vi "Main example.vi"() -> ()   [LabVIEW 2020]
uses:
  Control PaP/Support/Move motor.ctl
  Public/Controls/Command to motor.ctl
  Example States.ctl
  Control PaP/Support/Channel configuration--cluster.ctl
  Control PaP/Libraries/NI DAQ/NI DAQ.lvlib
  Control PaP/Libraries/TDS1002 Oscilloscope/TDS1002 Oscilloscope.lvlib
  <resource>/objmgr/daqmx.rc
  Control de MaP.lvlib
panel:
  in  "Motor params":T1={"Tipo"=0, "Dirección"=0, "N°. Pasos"=200, "Frecuencia (Hz)"=255, "Tipo de paso"=1} caption="Parámetros del motor" {"Tipo de paso" items=["Medio paso", "Paso completo"]; "Dirección" items=["Izquierda", "Derecha"]; "Tipo" items=["Unipolar", "Bipolar"]}
  out "Waveform Graph":waveform(dbl)(graph)
  in  "Mover motor":T2
  in  "Driver de motor":refnum<visa-resource-name>
  in  "Osciloscopio":refnum<visa-resource-name>
  in  "DAQ":u16(ring) items=["DAQ_Simulada", "Dev1"]
  in  "stop":bool
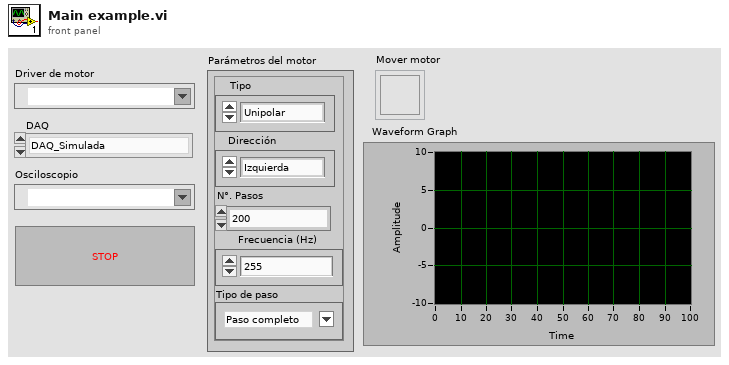
[diagram p1: front panel]
types:
  T1 = typedef "Control de MaP.lvlib/Command to motor.ctl" = cluster{"Tipo":u8, "Dirección":u8, "N°. Pasos":u16, "Frecuencia (Hz)":u8, "Tipo de paso":u8}
  T2 = typedef "Move motor.ctl" = bool
  T3 = cluster{"Driver de motor":refnum<visa-resource-name>, "DAQ ID":i32, "TDS ID":i32}
  T4 = typedef "Example States.ctl" = enum16{"Wait", "Initialize", "Exit"}
  T5 = typedef "TDS1002 Oscilloscope.lvlib/Broadcast Events--cluster.ctl" = cluster{"Module Did Init":refnum<user-event>, "Status Updated":refnum<user-event>, "Error Reported":refnum<user-event>, "Module Did Stop":refnum<user-event>, "Update Module Execution Status":refnum<user-event>, "Helper Loop Status Updated":refnum<user-event>, "Device connected":refnum<user-event>, "Device disconnected":refnum<user-event>, "Data acquired":refnum<user-event>}
  T6 = typedef "NI DAQ.lvlib/Broadcast Events--cluster.ctl" = cluster{"Module Did Init":refnum<user-event>, "Status Updated":refnum<user-event>, "Error Reported":refnum<user-event>, "Module Did Stop":refnum<user-event>, "Update Module Execution Status":refnum<user-event>, "Data acquired":refnum<user-event>}
  T7 = enum16{"All", "DO task", "DI task", "AO task", "AI task"}
  T8 = typedef "TDS1002 Oscilloscope.lvlib/Channel configuration--cluster.ctl" = cluster{"Acquisition Type":i32, "Averaged Waveforms":i32, "Channel":i32, "Probe Attenuation":i32}
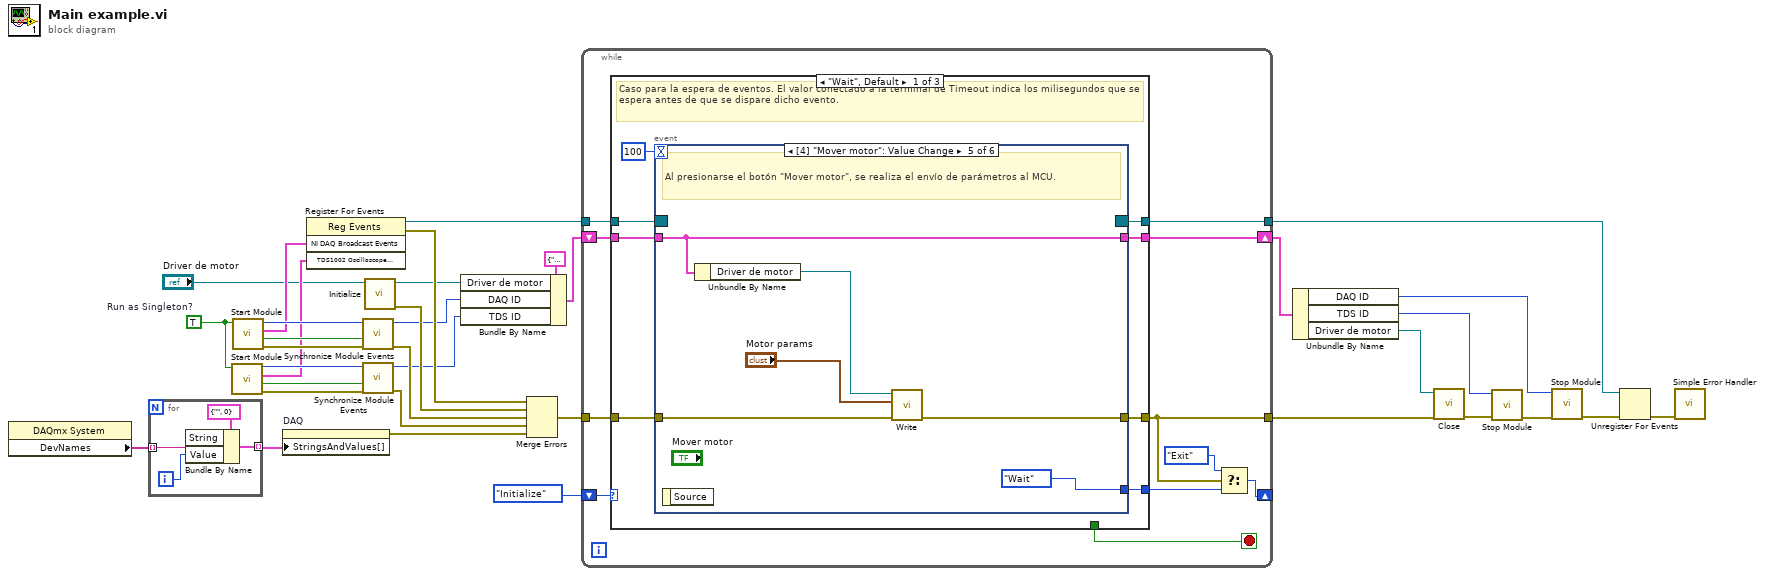
[diagram p0: block diagram]
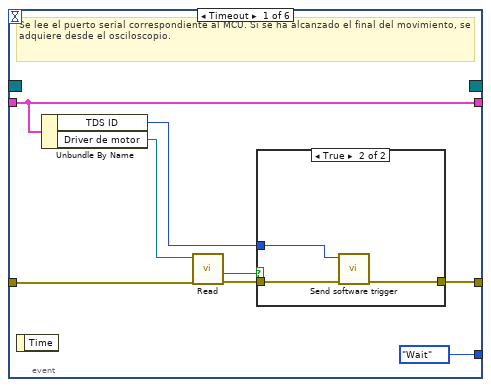
[diagram p2: hidden frame]
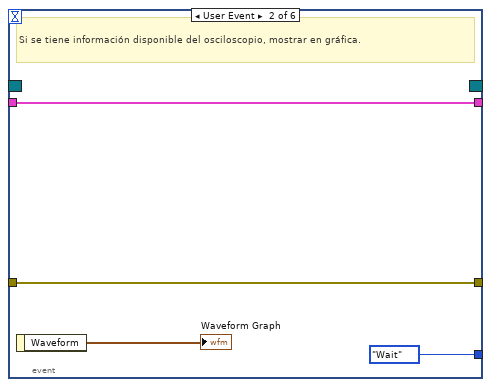
[diagram p4: hidden frame]
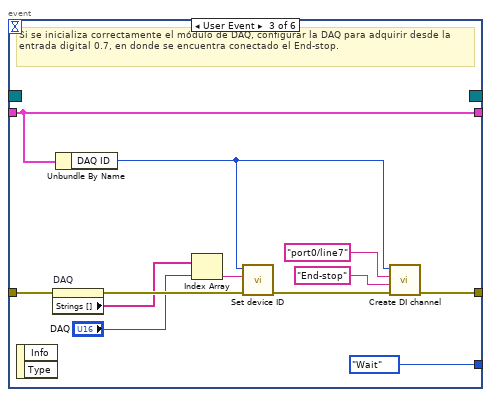
[diagram p5: hidden frame]
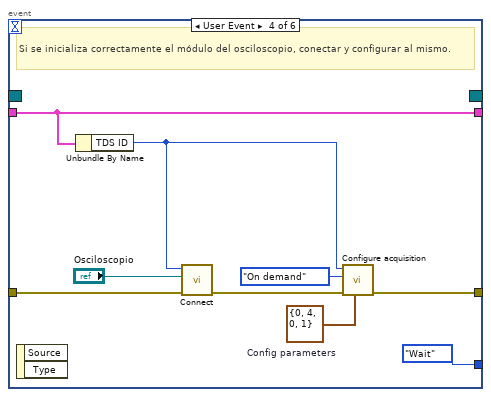
[diagram p6: hidden frame]
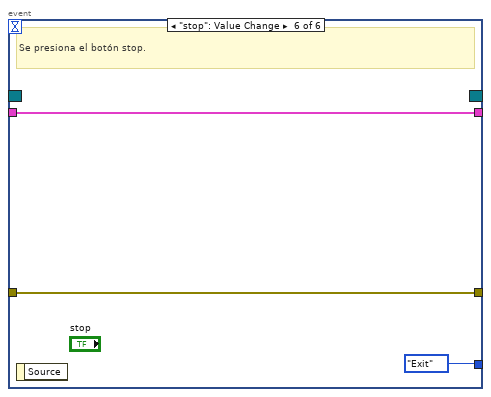
[diagram p7: hidden frame]
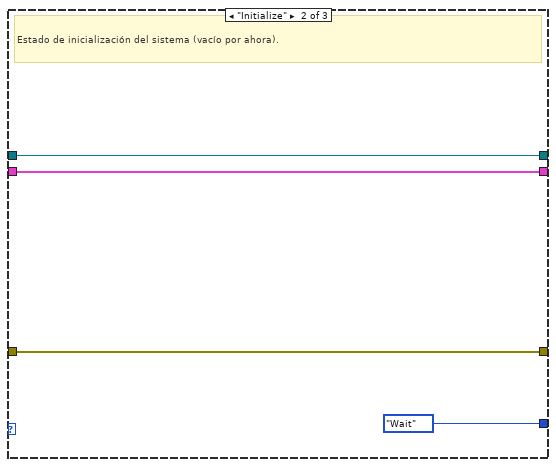
[diagram p8: hidden frame]
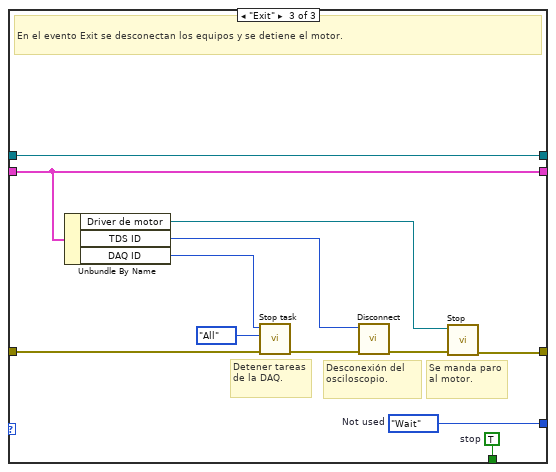
[diagram p9: hidden frame]
diagram:
  w23 = TRUE  # Run as Singleton?
  n1 = property class="DAQmx System"() -> ("DevNames"=w2:tag[])  [unwired: 2 in, 2 out]
  n2 = for {
    tunnel: w2 -> [w38] mode=indexing
    tunnel: [w36] -> w3 mode=indexing
    i -> [w37]
    n3 = Bundle By Name(cluster=cluster{"String":string, "Value":u16} {"String"="", "Value"=0} ("Cluster"), "String"=w38, "Value"=w37) -> (w36:cluster{"String":string, "Value":u16})
  }
  n4 = call "Start Module.vi"("Run as Singleton? (F)"=w23) -> ("error out"=w32:errorcluster, "Wait for Event Sync?"=w30:bool, "TDS1002 Oscilloscope Broadcast Events"=w28:T5, "Module ID"=w31:i32)  [unwired: 7 in]
  n5 = call "Start Module.vi"("Run as Singleton? (F)"=w23) -> ("error out"=w35:errorcluster, "Wait for Event Sync?"=w33:bool, "NI DAQ Broadcast Events"=w29:T6, "Module ID"=w34:i32)  [unwired: 7 in]
  n6 = property on="DAQ" class="Ring (strict)"("StringsAndValues[]"=w3) -> (error out=w1:errorcluster)  [unwired: 2 in, 1 out]
  n7 = register-events(w29, w28) -> (reference out=w20:refnum<event-registration>, error out=w25:errorcluster)  [unwired: 2 in]
  n8 = call "Synchronize Module Events.vi"("error in"=w35, "Wait for Event Sync?"=w33, "Module ID in"=w34) -> ("error out"=w26:errorcluster, "Module ID out"=w12:i32)  [unwired: 7 in]
  n9 = call "Synchronize Module Events.vi"("error in"=w32, "Wait for Event Sync?"=w30, "Module ID in"=w31) -> ("error out"=w27:errorcluster, "Module ID out"=w11:i32)  [unwired: 7 in]
  n10 = call "Initialize.vi"("Puerto Serial"="Driver de motor") -> ("error out"=w16:errorcluster, "VISA resource name out"=w14:refnum<visa-resource-name>)  [unwired: 9 in]
  n11 = Bundle By Name(cluster=T3 {"Driver de motor"="", "DAQ ID"=0, "TDS ID"=0} ("Data"), "Driver de motor"=w14, "DAQ ID"=w12, "TDS ID"=w11) -> (w10:T3)
  n12 = Merge Errors(w25, w16, w26, w27, w1) -> (w24:errorcluster)
  n13 = while {
    tunnel: w24 -> [w50]
    tunnel: [w41] -> w7
    shift-right: [w42] -> _
    shift-left: Example_States."Initialize" -> [w48]
    tunnel: w20 -> [w47]
    tunnel: [w46] -> w18
    shift-right: [w45] -> w9
    shift-left: w10 -> [w44]
    stop <- w49 stop-if-true
    n14 = case shown="\"Wait\", Default" w48 {
      tunnel: w50 -> [w58 w105 w117]
      tunnel: [w57 w105 w110] -> w41
      tunnel: [_ _ w119] -> w49
      tunnel: [w56 Example_States."Wait" ("Not used") w115] -> w43
      tunnel: w47 -> [w55 w107 w120]
      tunnel: [w54 w107 w120] -> w46
      tunnel: [w51 w106 w114] -> w45
      tunnel: w44 -> [w52 w106 w114]
      frame "Wait", Default {
        # "Caso para la espera de eventos. El valor conectado a la terminal de Timeout indica los milisegundos que se espera antes de que se dispare dicho evento."
        n15 = event shown="[4] \"Mover motor\": Value Change" {
          selector: w55 -> [_ _ _ _ _ _]
          dyn-events: [_ _ _ _ _ _] -> w54
          timeout: 100 -> [_ _ _ _ _ _]
          tunnel: w58 -> [w65 w73 w86 w95 w100 w104]
          tunnel: [w60 w73 w81 w91 w99 w104] -> w57
          tunnel: [Example_States."Wait" ("Not used") Example_States."Wait" Example_States."Wait" Example_States."Wait" Example_States."Wait" Example_States."Exit"] -> w56
          tunnel: w52 -> [w64 w74 w78 w88 w98 w102]
          tunnel: [w64 w74 w78 w88 w98 w102] -> w51
          event Timeout {
            # "Se lee el puerto serial correspondiente al MCU. Si se ha alcanzado el final del movimiento, se adquiere desde el osciloscopio."
            n16 = event-data() -> ()  [unwired: 1 in, 1 out]
            n17 = Unbundle By Name(w64) -> ("TDS ID"=w59:i32, "Driver de motor"=w63:refnum<visa-resource-name>)
            n18 = call "Read.vi"("error in (no error)"=w65, "VISA resource name"=w63) -> ("error out"=w61:errorcluster, "End"=w62:bool)  [unwired: 6 in, 2 out]
            n19 = case shown="True" w62 {
              tunnel: w61 -> [w67 w70]
              tunnel: [w67 w69] -> w60
              tunnel: w59 -> [_ w68]
              frame False {
              }
              frame True {
                n20 = call "Send software trigger.vi"("error in"=w70, "Module ID"=w68) -> ("error out"=w69:errorcluster)  [unwired: 9 in]
              }
            }
          }
          event User Event {
            # "Si se tiene información disponible del osciloscopio, mostrar en gráfica."
            n21 = event-data() -> ("Waveform"=→"Waveform Graph":waveform(dbl))  [unwired: 1 in]
          }
          event User Event {
            # "Si se inicializa correctamente el módulo de DAQ, configurar la DAQ para adquirir desde la entrada digital 0.7, en donde se encuentra conectado el End-stop."
            n22 = event-data() -> ()  [unwired: 1 in, 2 out]
            n23 = property on="DAQ" class="Ring (strict)"(error in=w86) -> (error out=w85:errorcluster, "Strings []"=w84:string[])  [unwired: 1 in, 1 out]
            n24 = Unbundle By Name(w78) -> ("DAQ ID"=w77:i32)
            n25 = Index Array(array=w84, index="DAQ") -> (element=w83:string)
            n26 = call "Set device ID.vi"("error in"=w85, "Device ID"=w83, "Module ID"=w77) -> ("error out"=w82:errorcluster)  [unwired: 8 in]
            n27 = call "Create DI channel.vi"("error in"=w82, "Channel name"="End-stop", "Physical channel"="port0/line7", "Module ID"=w77) -> ("error out"=w81:errorcluster)  [unwired: 7 in]
          }
          event User Event {
            w92 = T8 {"Acquisition Type"=0, "Averaged Waveforms"=4, "Channel"=0, "Probe Attenuation"=1}  # Config parameters
            # "Si se inicializa correctamente el módulo del osciloscopio, conectar y configurar al mismo."
            n28 = event-data() -> ()  [unwired: 1 in, 2 out]
            n29 = Unbundle By Name(w88) -> ("TDS ID"=w87:i32)
            n30 = call "Connect.vi"("error in"=w95, "VISA resource name"="Osciloscopio", "Module ID"=w87) -> ("error out"=w94:errorcluster)  [unwired: 8 in]
            n31 = call "Configure acquisition.vi"("Config parameters"=w92, "error in"=w94, "Type"=enum16{"On demand", "Continous"}."On demand", "Module ID"=w87) -> ("error out"=w91:errorcluster)  [unwired: 7 in]
          }
          event Value Change {
            # "Al presionarse el botón \"Mover motor\", se realiza el envío de parámetros al MCU."
            n32 = event-data() -> ()  [unwired: 1 in, 1 out]
            n33 = Unbundle By Name(w98) -> ("Driver de motor"=w97:refnum<visa-resource-name>)
            n34 = call "Write.vi"("error in (no error)"=w100, "Comando"="Motor params", "VISA resource name"=w97) -> ("error out"=w99:errorcluster)  [unwired: 6 in, 2 out]
          }
          event "stop": Value Change {
            # "Se presiona el botón stop."
            n35 = event-data() -> ()  [unwired: 1 in, 1 out]
          }
        }
      }
      frame "Initialize" {
        # "Estado de inicialización del sistema (vacío por ahora)."
      }
      frame "Exit" {
        w115 = Example_States."Wait"  # Not used
        w119 = TRUE  # stop
        # "Se manda paro al motor."
        # "Desconexión del osciloscopio."
        # "Detener tareas de la DAQ."
        # "En el evento Exit se desconectan los equipos y se detiene el motor."
        n36 = Unbundle By Name(w114) -> ("Driver de motor"=w109:refnum<visa-resource-name>, "TDS ID"=w112:i32, "DAQ ID"=w113:i32)
        n37 = call "Stop task.vi"("error in"=w117, "Task list"=T7."All", "Module ID"=w113) -> ("error out"=w118:errorcluster)  [unwired: 8 in]
        n38 = call "Disconnect.vi"("error in"=w118, "Module ID"=w112) -> ("error out"=w111:errorcluster)  [unwired: 9 in]
        n39 = call "Stop.vi"("error in (no error)"=w111, "VISA resource name"=w109) -> ("error out"=w110:errorcluster)  [unwired: 8 in, 1 out]
      }
    }
    n40 = Select(t=Example_States."Exit", s=w41, f=w43) -> (s? t:f=w42:T4)
  }
  n41 = Unbundle By Name(w9) -> ("DAQ ID"=w4:i32, "TDS ID"=w5:i32, "Driver de motor"=w6:refnum<visa-resource-name>)
  n42 = call "Close.vi"("error in (no error)"=w7, "VISA resource name"=w6) -> ("error out"=w8:errorcluster)  [unwired: 9 in]
  n43 = call "Stop Module.vi"("error in"=w8, "Module ID"=w5) -> ("error out"=w22:errorcluster)  [unwired: 9 in]
  n44 = call "Stop Module.vi"("error in"=w22, "Module ID"=w4) -> ("error out"=w19:errorcluster)  [unwired: 9 in]
  n45 = Unregister For Events(event registration refnum=w18, error in=w19) -> (error out=w17:errorcluster)
  n46 = call <vilib>:"Simple Error Handler.vi"("error in (no error)"=w17) -> ()  [unwired: 4 in, 5 out]
